vi "Keithley 2600 Series Control Toggle Channel B.vi"() -> ()   [LabVIEW 2017]
doc: "This example shows how to configure the source output and perform multiple current measurements."
uses:
  <instrlib>/Keithley 2600 Series/Keithley 2600 Series.lvlib
panel:
  in  "Aperture State":u16(ring) items=["Always OFF", "Always ON", "ON During Sweep OFF Otherwise", "OFF During Sweep ON Otherwise"]
  in  "Inter Sweep Delay(ms)":dbl
  in  "VISA resource name":refnum<visa-resource-name>
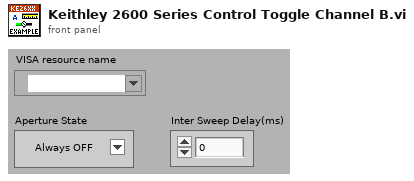
[diagram p1: front panel]
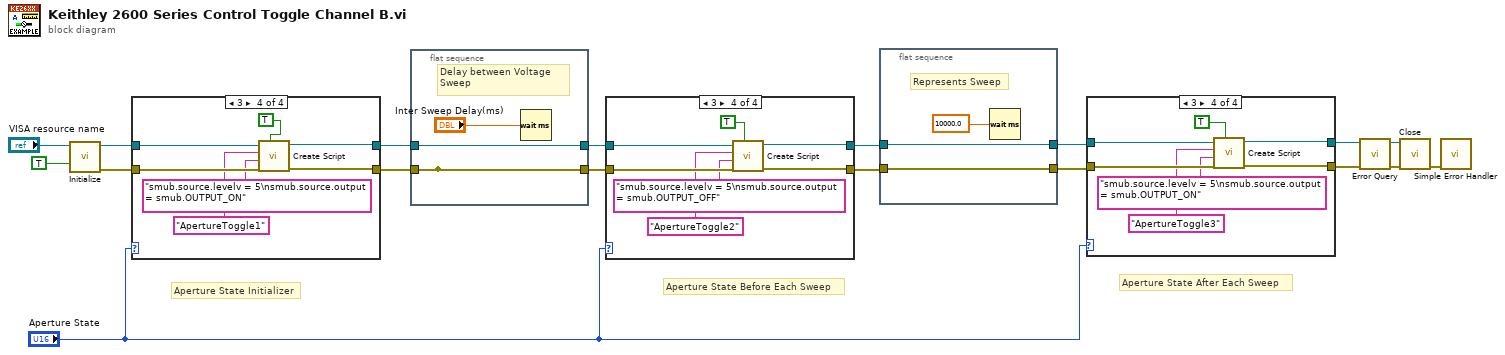
[diagram p0: block diagram]
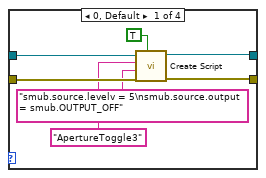
[diagram p2: hidden frame]
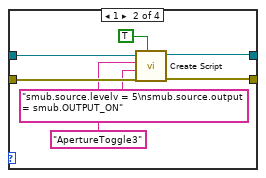
[diagram p3: hidden frame]
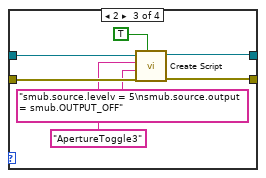
[diagram p4: hidden frame]
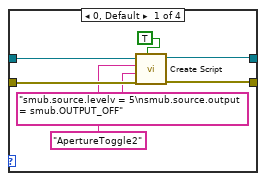
[diagram p5: hidden frame]
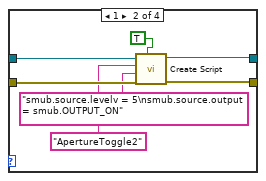
[diagram p6: hidden frame]
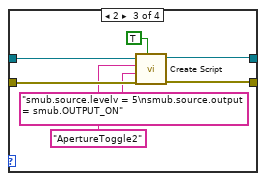
[diagram p7: hidden frame]
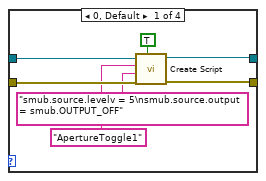
[diagram p8: hidden frame]
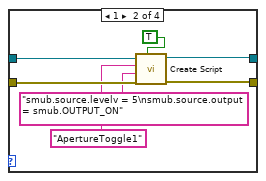
[diagram p9: hidden frame]
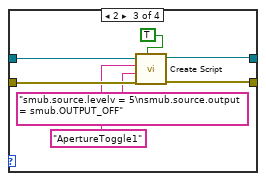
[diagram p10: hidden frame]
diagram:
  # "Aperture State Before Each Sweep"
  # "Aperture State After Each Sweep"
  # "Aperture State Initializer"
  n1 = call <instrlib>:"Initialize.vi"("Reset (True)"=TRUE, "VISA resource name"="VISA resource name") -> ("error out"=w15:errorcluster, "VISA resource name out"=w16:refnum<visa-resource-name>)  [unwired: 8 in]
  n2 = case shown="3" "Aperture State" {
    tunnel: w16 -> [w25 w32 w39 w46]
    tunnel: w15 -> [w22 w29 w36 w43]
    tunnel: [w24 w31 w38 w45] -> w14
    tunnel: [w23 w30 w37 w44] -> w13
    frame 0, Default {
      n3 = call <instrlib>:"Create Script.vi"("Auto Run (F: Disable)"=TRUE, "error in (no error)"=w22, "Source Code"="smub.source.levelv = 5\nsmub.source.output = smub.OUTPUT_OFF", "Script Variable"="ApertureToggle1", "VISA resource name"=w25) -> ("error out"=w23:errorcluster, "VISA resource name out"=w24:refnum<visa-resource-name>)  [unwired: 5 in]
    }
    frame 1 {
      n4 = call <instrlib>:"Create Script.vi"("Auto Run (F: Disable)"=TRUE, "error in (no error)"=w29, "Source Code"="smub.source.levelv = 5\nsmub.source.output = smub.OUTPUT_ON", "Script Variable"="ApertureToggle1", "VISA resource name"=w32) -> ("error out"=w30:errorcluster, "VISA resource name out"=w31:refnum<visa-resource-name>)  [unwired: 5 in]
    }
    frame 2 {
      n5 = call <instrlib>:"Create Script.vi"("Auto Run (F: Disable)"=TRUE, "error in (no error)"=w36, "Source Code"="smub.source.levelv = 5\nsmub.source.output = smub.OUTPUT_OFF", "Script Variable"="ApertureToggle1", "VISA resource name"=w39) -> ("error out"=w37:errorcluster, "VISA resource name out"=w38:refnum<visa-resource-name>)  [unwired: 5 in]
    }
    frame 3 {
      n6 = call <instrlib>:"Create Script.vi"("Auto Run (F: Disable)"=TRUE, "error in (no error)"=w43, "Source Code"="smub.source.levelv = 5\nsmub.source.output = smub.OUTPUT_ON", "Script Variable"="ApertureToggle1", "VISA resource name"=w46) -> ("error out"=w44:errorcluster, "VISA resource name out"=w45:refnum<visa-resource-name>)  [unwired: 5 in]
    }
  }
  n7 = flat-sequence {
    tunnel: w14 -> [w49]
    tunnel: w13 -> [w47]
    tunnel: [w47] -> _
    tunnel: [w49] -> w9
    tunnel: [w47] -> w8
    frame #0 {
      # "Delay between Voltage Sweep"
      n8 = Wait (ms)(milliseconds to wait="Inter Sweep Delay(ms)") -> ()  [unwired: 1 out]
    }
  }
  n9 = case shown="3" "Aperture State" {
    tunnel: w9 -> [w56 w63 w70 w77]
    tunnel: w8 -> [w53 w60 w67 w74]
    tunnel: [w55 w62 w69 w76] -> w7
    tunnel: [w54 w61 w68 w75] -> w6
    frame 0, Default {
      n10 = call <instrlib>:"Create Script.vi"("Auto Run (F: Disable)"=TRUE, "error in (no error)"=w53, "Source Code"="smub.source.levelv = 5\nsmub.source.output = smub.OUTPUT_OFF", "Script Variable"="ApertureToggle2", "VISA resource name"=w56) -> ("error out"=w54:errorcluster, "VISA resource name out"=w55:refnum<visa-resource-name>)  [unwired: 5 in]
    }
    frame 1 {
      n11 = call <instrlib>:"Create Script.vi"("Auto Run (F: Disable)"=TRUE, "error in (no error)"=w60, "Source Code"="smub.source.levelv = 5\nsmub.source.output = smub.OUTPUT_ON", "Script Variable"="ApertureToggle2", "VISA resource name"=w63) -> ("error out"=w61:errorcluster, "VISA resource name out"=w62:refnum<visa-resource-name>)  [unwired: 5 in]
    }
    frame 2 {
      n12 = call <instrlib>:"Create Script.vi"("Auto Run (F: Disable)"=TRUE, "error in (no error)"=w67, "Source Code"="smub.source.levelv = 5\nsmub.source.output = smub.OUTPUT_ON", "Script Variable"="ApertureToggle2", "VISA resource name"=w70) -> ("error out"=w68:errorcluster, "VISA resource name out"=w69:refnum<visa-resource-name>)  [unwired: 5 in]
    }
    frame 3 {
      n13 = call <instrlib>:"Create Script.vi"("Auto Run (F: Disable)"=TRUE, "error in (no error)"=w74, "Source Code"="smub.source.levelv = 5\nsmub.source.output = smub.OUTPUT_OFF", "Script Variable"="ApertureToggle2", "VISA resource name"=w77) -> ("error out"=w75:errorcluster, "VISA resource name out"=w76:refnum<visa-resource-name>)  [unwired: 5 in]
    }
  }
  n14 = flat-sequence {
    tunnel: w7 -> [w79]
    tunnel: w6 -> [w80]
    tunnel: [w80] -> w2
    tunnel: [w79] -> w3
    frame #0 {
      # "Represents Sweep"
      n15 = Wait (ms)(milliseconds to wait=10000.0 ("Inter Sweep Delay(ms) 2")) -> ()  [unwired: 1 out]
    }
  }
  n16 = case shown="3" "Aperture State" {
    tunnel: w3 -> [w87 w94 w101 w108]
    tunnel: w2 -> [w84 w91 w98 w105]
    tunnel: [w86 w93 w100 w107] -> w5
    tunnel: [w85 w92 w99 w106] -> w4
    frame 0, Default {
      n17 = call <instrlib>:"Create Script.vi"("Auto Run (F: Disable)"=TRUE, "error in (no error)"=w84, "Source Code"="smub.source.levelv = 5\nsmub.source.output = smub.OUTPUT_OFF", "Script Variable"="ApertureToggle3", "VISA resource name"=w87) -> ("error out"=w85:errorcluster, "VISA resource name out"=w86:refnum<visa-resource-name>)  [unwired: 5 in]
    }
    frame 1 {
      n18 = call <instrlib>:"Create Script.vi"("Auto Run (F: Disable)"=TRUE, "error in (no error)"=w91, "Source Code"="smub.source.levelv = 5\nsmub.source.output = smub.OUTPUT_ON", "Script Variable"="ApertureToggle3", "VISA resource name"=w94) -> ("error out"=w92:errorcluster, "VISA resource name out"=w93:refnum<visa-resource-name>)  [unwired: 5 in]
    }
    frame 2 {
      n19 = call <instrlib>:"Create Script.vi"("Auto Run (F: Disable)"=TRUE, "error in (no error)"=w98, "Source Code"="smub.source.levelv = 5\nsmub.source.output = smub.OUTPUT_OFF", "Script Variable"="ApertureToggle3", "VISA resource name"=w101) -> ("error out"=w99:errorcluster, "VISA resource name out"=w100:refnum<visa-resource-name>)  [unwired: 5 in]
    }
    frame 3 {
      n20 = call <instrlib>:"Create Script.vi"("Auto Run (F: Disable)"=TRUE, "error in (no error)"=w105, "Source Code"="smub.source.levelv = 5\nsmub.source.output = smub.OUTPUT_ON", "Script Variable"="ApertureToggle3", "VISA resource name"=w108) -> ("error out"=w106:errorcluster, "VISA resource name out"=w107:refnum<visa-resource-name>)  [unwired: 5 in]
    }
  }
  n21 = call <instrlib>:"Error Query.vi"("error in (no error)"=w4, "VISA resource name"=w5) -> ("error out"=w10:errorcluster, "VISA resource name out"=w11:refnum<visa-resource-name>)  [unwired: 6 in, 2 out]
  n22 = call <instrlib>:"Close.vi"("error in (no error)"=w10, "VISA resource name"=w11) -> ("error out"=w12:errorcluster)  [unwired: 9 in]
  n23 = call <vilib>:"Simple Error Handler.vi"("error in (no error)"=w12) -> ()  [unwired: 4 in, 5 out]
